vi "VeriStand DSF.Transfer.Configuration.Verify.Channels Configuration.vi"(8 "error in (no error)":errorcluster, 11 "channel configurations":T1[](array[typedef])) -> (0 "error out":errorcluster)   [LabVIEW 2017, in "Data Sharing Custom Device Engine.lvlib" / "VeriStand DSF.Transfer.Configuration.lvclass"]
uses:
  VeriStand DSF.Transfer.Configuration.lvclass
  Builds/Data Sharing Framework/Current/Data Sharing Framework Core/DSF Core.lvlibp/DSF Configuration API/Public/Controls/DSF Engine Channel Configuration.ctl
  Builds/Data Sharing Framework/Current/Data Sharing Framework Core/DSF Core.lvlibp/DSF Configuration API/Public/Controls/DSF Data Type.ctl
  Builds/Data Sharing Framework/Current/Data Sharing Framework Core/DSF Core.lvlibp/DSF Configuration API/Public/Controls/DSF Settings Info.ctl
  Builds/Data Sharing Framework/Current/Data Sharing Framework Core/DSF Core.lvlibp
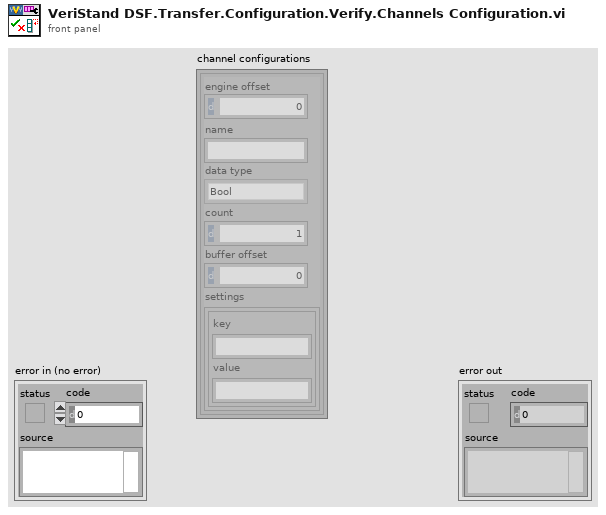
[diagram p1: front panel]
types:
  T1 = typedef "DSF Core.lvlibp/DSF Engine Channel Configuration.ctl" = cluster{"engine offset":u64, "name":string, "data type":T2, "count":u64, "buffer offset":u64, "settings":T3}
  T2 = typedef "DSF Core.lvlibp/DSF Data Type.ctl" = enum8{"Bool", "SGL", "DBL", "I8", "I16", "I32", "I64", "U8", "U16", "U32", "U64"}
  T3 = typedef "DSF Core.lvlibp/DSF Settings Info.ctl" = cluster{"key":string, "value":string}[]
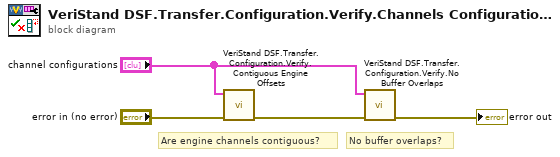
[diagram p0: block diagram]
diagram:
  # "No buffer overlaps?"
  # "Are engine channels contiguous?"
  n1 = call "VeriStand DSF.Transfer.Configuration.Verify.Contiguous Engine Offsets.vi"("error in (no error)"="error in (no error)", "channel configurations"="channel configurations") -> ("error out"=w3:errorcluster)  [unwired: 9 in]
  n2 = call "VeriStand DSF.Transfer.Configuration.Verify.No Buffer Overlaps.vi"("error in (no error)"=w3, "channel configurations"="channel configurations") -> ("error out"=→"error out":errorcluster)  [unwired: 9 in]
